vi "Check Active Window.vi"(3 "Filename":string) -> (1 "Active Window":bool)   [LabVIEW 2013]
uses:
  USER32.DLL
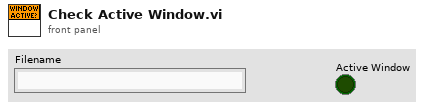
[diagram p1: front panel]
types:
  T1 = cluster{"cbSize":i32, "rcWindow":cluster{"left":i32, "top":i32, "right":i32, "bottom":i32}, "rcClient":cluster{"left":i32, "top":i32, "right":i32, "bottom":i32}, "dwStyle":i32, "dwExStyle":i32, "dwWindowStatus":i32, "cxWindowBorders":u32, "cyWindowBorders":u32, "atomWindowType":u16, "wCreatorVersion":u16}
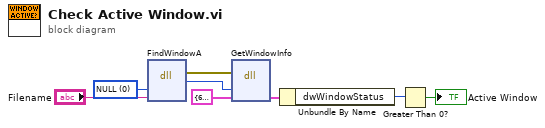
[diagram p0: block diagram]
diagram:
  w8 = 0 items=["NULL"]
  n1 = dll-call lib="user32.dll" fn="FindWindowA"("lpClassName"=w8, "lpWindowName"="Filename") -> (error out=w4:errorcluster, "hWnd"=w3:i32)  [unwired: 5 in, 1 out]
  n2 = dll-call lib="user32.dll" fn="GetWindowInfo"(error in=w4, "hWnd"=w3, "pwi"=T1 {"cbSize"=60, "rcWindow"={"left"=0, "top"=0, "right"=0, "bottom"=0}, "rcClient"={"left"=0, "top"=0, "right"=0, "bottom"=0}, "dwStyle"=0, "dwExStyle"=0, "dwWindowStatus"=0, "cxWindowBorders"=0, "cyWindowBorders"=0, "atomWindowType"=0, "wCreatorVersion"=0}) -> ("pwi"=w1:T1)  [unwired: 4 in, 2 out]
  n3 = Unbundle By Name(w1) -> ("dwWindowStatus"=w5:i32)
  n4 = Greater Than 0?(x=w5) -> (x > 0?=→"Active Window":bool)
